vi "Direction.vi"(9 "pin":i32, 10 "handle":u32, 11 "Direction?":bool) -> (3 "Succés?":bool)   [LabVIEW 2020]
uses:
  cDaqlib/cDaq.lvlib
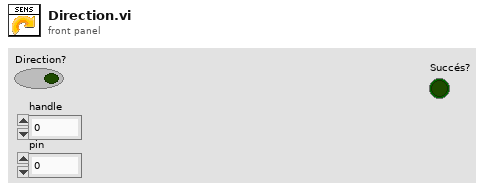
[diagram p1: front panel]
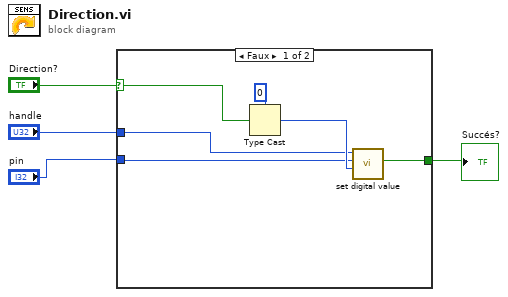
[diagram p0: block diagram]
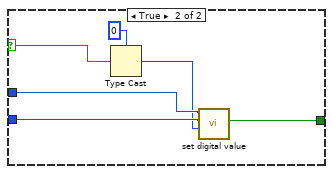
[diagram p2: hidden frame]
diagram:
  n1 = case shown="Faux" "Direction?" {
    selector: "Direction?" -> [w8 w14]
    tunnel: "handle" -> [w7 w16]
    tunnel: "pin" -> [w6 w15]
    tunnel: [w5 w11] -> w1
    frame False {
      n2 = Type Cast(type=0, x=w8) -> (*(type *) &x=w10:i32)
      n3 = call "set digital value .vi"("state"=w10, "pin"=w6, "handle"=w7) -> ("function return"=w5:bool)  [unwired: 7 in, 1 out]
    }
    frame True {
      n4 = Type Cast(type=0, x=w14) -> (*(type *) &x=w12:i32)
      n5 = call "set digital value .vi"("state"=w12, "pin"=w15, "handle"=w16) -> ("function return"=w11:bool)  [unwired: 7 in, 1 out]
    }
  }
  "Succés?" <- w1
